vi "Test Harness.vi"() -> ()   [LabVIEW 2020]
uses:
  Test Results.ctl
  12e9b78b-923a-47b1-88eb-dff865da94a5.vi
panel:
  out "Results":T1[](array[typedef])
  out "error out":errorcluster
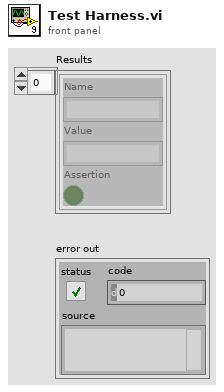
[diagram p1: front panel]
types:
  T1 = typedef "Test Results.ctl" = cluster{"Name":string, "Value":string, "Assertion":bool}
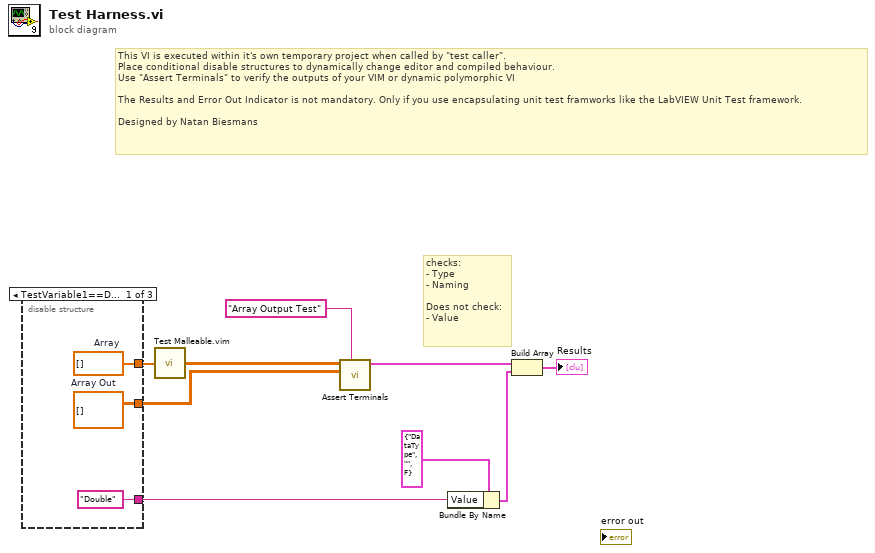
[diagram p0: block diagram]
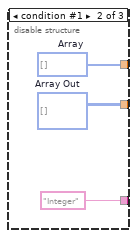
[diagram p2: hidden frame]
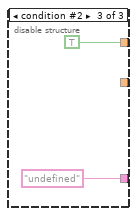
[diagram p3: hidden frame]
diagram:
  # "This VI is executed within it's own temporary project when called by \"test caller\".\nPlace conditional disable structures to dynamically change editor and compiled behaviour.\nUse \"Assert Terminals\" to verify the outputs of your VIM or dynamic polymorphic VI\n\nThe Results and Error Out Indicator is not mandatory. Only if you use encapsulating unit test framworks like the LabVIEW Unit Test framework.\n\nDesigned by Natan Biesmans"
  # "checks:\n- Type\n- Naming\n\nDoes not check:\n- Value"
  n1 = disable-structure shown="TestVariable1==Double" {
    disable-tunnel: [w12 w15 TRUE] -> w9
    disable-tunnel: [w11 w14 _] -> w3
    disable-tunnel: ["Double" ("Value") "Integer" ("Value") "undefined" ("Value")] -> w5
    frame condition #0 (active) {
      w11 = dbl[][] []  # Array Out
      w12 = dbl[] []  # Array
    }
    frame condition #1 {
      w14 = i16[][] []  # Array Out
      w15 = i16[] []  # Array
    }
    frame condition #2 {
    }
  }
  n2 = call "Test Malleable.vim"("Array"=w9) -> ("Array Out"=w4:dbl[][])
  n3 = call "Assert Terminals.vi"("Name"="Array Output Test", "Value in 2"=w3, "Value in 1"=w4) -> ("Assertion Result"=w2:T1)  [unwired: 7 in, 1 out]
  n4 = Bundle By Name(cluster=T1 {"Name"="DataType", "Value"="", "Assertion"=FALSE} ("Cluster"), "Value"=w5) -> (w6:T1)
  n5 = Build Array(w2, w6) -> (→"Results":T1[])
